vi "2static.vi"() -> ()   [LabVIEW 2026]
panel:
  in  "OK Button 3":bool
  in  "OK Button 2":bool
  in  "OK Button":bool
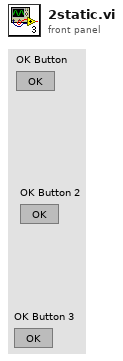
[diagram p1: front panel]
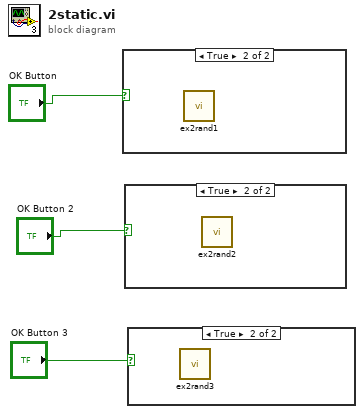
[diagram p0: block diagram]
diagram:
  n1 = case shown="True" "OK Button" {
    frame False {
    }
    frame True {
      n2 = call "ex2rand1.vi"() -> ()  [unwired: 12 in]
    }
  }
  n3 = case shown="True" "OK Button 2" {
    frame False {
    }
    frame True {
      n4 = call "ex2rand2.vi"() -> ()  [unwired: 12 in]
    }
  }
  n5 = case shown="True" "OK Button 3" {
    frame False {
    }
    frame True {
      n6 = call "ex2rand3.vi"() -> ()  [unwired: 12 in]
    }
  }
